vi "Define Home.vi"(8 "error in (no error)":errorcluster, 9 "Home (Unit/s)":dbl, 10 "Axis":i32=1, 11 "VISA resource name in":refnum<visa-resource-name>) -> (0 "error out":errorcluster, 3 "VISA resource name out":refnum<visa-resource-name>)   [LabVIEW 2019]
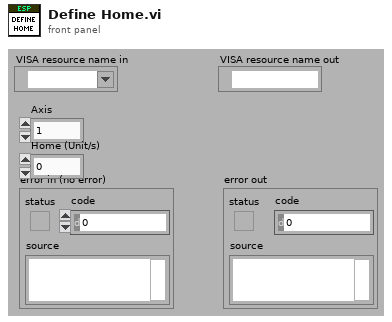
[diagram p1: front panel]
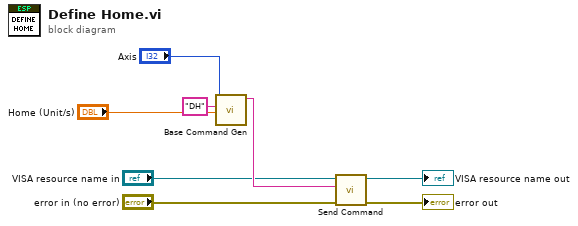
[diagram p0: block diagram]
diagram:
  n1 = call "Base Command Gen.vi"("nn1"="Home (Unit/s)", "Command"="DH", "xx"="Axis") -> ("Command"=w5:string)  [unwired: 8 in]
  n2 = call "Send Command.vi"("error out (no error)"="error in (no error)", "Command"=w5, "VISA resource name in"="VISA resource name in") -> ("error out"=→"error out":errorcluster, "VISA resource name out"=→"VISA resource name out":refnum<visa-resource-name>)  [unwired: 7 in]
